vi "Test Find Shortest.vi"(11 "Test Case In":refnum<class "Directional Keypad Test.lvclass">) -> (0 "error out":errorcluster, 3 "Test Case Out":refnum<class "Directional Keypad Test.lvclass">)   [LabVIEW 2020, in "Directional Keypad Test.lvclass"]
uses:
  Directional Keypad Test.lvclass
  C:/Program Files (x86)/National Instruments/LabVIEW 2020/vi.lib/Astemes/LUnit/Test Case.lvclass
  Directional Keypad Test.lvclass/Directional Keypad Test.ctl
  <vilib>/Astemes/LUnit/Test Case.lvclass/Test Case.ctl
  7c7748cc-d5ce-4aad-accd-a52b5d69d203.vi
  <vilib>/Astemes/LUnit/Palette/Pass If.vi
  <vilib>/Astemes/LUnit/Append Fail Result.vi
  <vilib>/Astemes/LUnit/Append Pass Result.vi
  <vilib>/Astemes/LUnit/Run In UI.vi
  <vilib>/Utility/error.llb/Clear Errors.vi
  Directional Keypad/Directional Keypad.lvclass
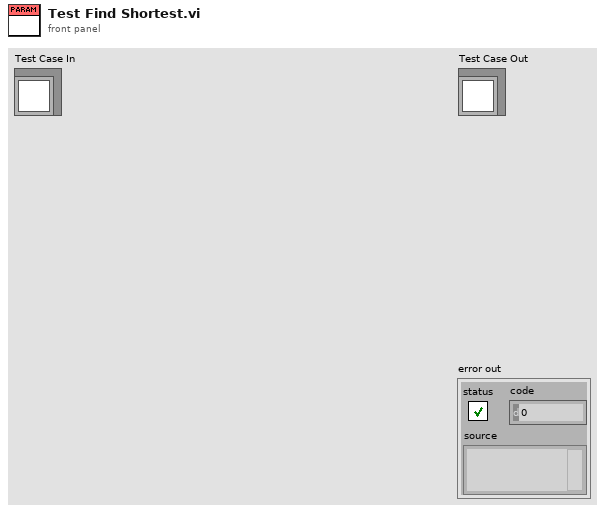
[diagram p1: front panel]
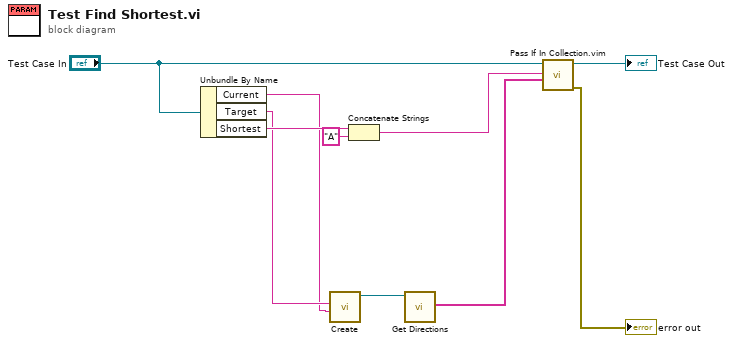
[diagram p0: block diagram]
diagram:
  n1 = Unbundle By Name("Test Case In") -> ("Current"=w3:string, "Target"=w4:string, "Shortest"=w6:string)
  n2 = call "Create.vi"("Current"=w3, "Input"=w4) -> ("Proto"=w7:refnum<class "Directional Keypad.lvclass">)  [unwired: 9 in]
  n3 = Concatenate Strings(w6, "A" ("string")) -> (w2:string)
  n4 = call "Get Directions.vi"("Proto in"=w7) -> ("Directional Button Presses"=w5:string[])  [unwired: 9 in, 1 out]
  n5 = call "Pass If In Collection.vim"("Collection"=w5, "Expected Element"=w2, "LUnit Test Case In"="Test Case In") -> ("error out"=→"error out":errorcluster, "LUnit Test Case Out"=→"Test Case Out":refnum<class "Directional Keypad Test.lvclass">)  [unwired: 7 in]
